vi "Area.vi"(8 "error in (no error)":errorcluster caption="错误输入（无错误）", 11 "Size 输入":refnum<class "Size.lvclass"> caption="DNL_LabVIEW Object in") -> (0 "error out":errorcluster caption="错误输出", 2 "Area":dbl, 3 "Size 输出":refnum<class "Size.lvclass"> caption="DNL_LabVIEW Object out")   [LabVIEW 2011, in "Size.lvclass"]
uses:
  Size.lvclass
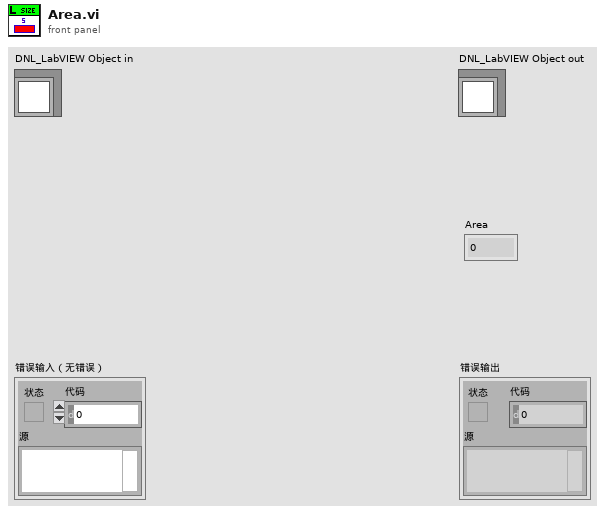
[diagram p1: front panel]
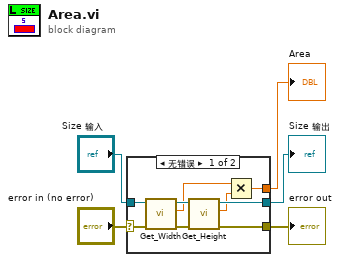
[diagram p0: block diagram]
diagram:
  n1 = case shown="无错误" "error in (no error)" {
    selector: "error in (no error)" -> [w8 w16]
    tunnel: [w6 w16] -> w4
    tunnel: [w12 w15] -> w2
    tunnel: "Size 输入" -> [w14 w15]
    tunnel: [w9 _] -> w1
    frame No Error {
      n2 = call "Get_Width.vi"("error in (no error)"=w8, "Size输入"=w14) -> ("error out"=w7:errorcluster, "Width"=w11:dbl, "Size输出"=w13:refnum<class "Size.lvclass">)  [unwired: 7 in]
      n3 = call "Get_Height.vi"("error in (no error)"=w7, "Size输入"=w13) -> ("error out"=w6:errorcluster, "Height"=w10:dbl, "Size输出"=w12:refnum<class "Size.lvclass">)  [unwired: 7 in]
      n4 = Multiply(x=w11, y=w10) -> (x*y=w9:dbl)
    }
    frame Error {
    }
  }
  "error out" <- w4
  "Size 输出" <- w2
  "Area" <- w1
